vi "Kalman_Filter_Initialize.vi"(8 "error in (no error)":errorcluster, 11 "Kalman_Filter in":refnum<class "Kalman_Filter.lvclass">) -> (0 "error out":errorcluster, 3 "Kalman_Filter out":refnum<class "Kalman_Filter.lvclass">)   [LabVIEW 2021, in "Kalman_Filter.lvclass"]
uses:
  Kalman_Filter.lvclass
  Kalman_Filter.lvclass/Kalman_Filter.ctl
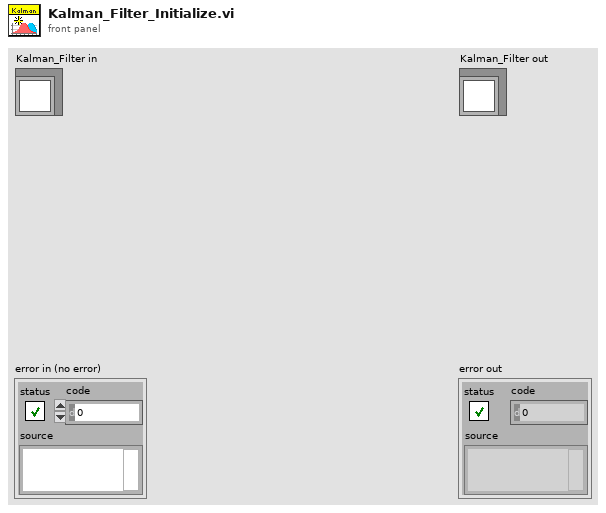
[diagram p1: front panel]
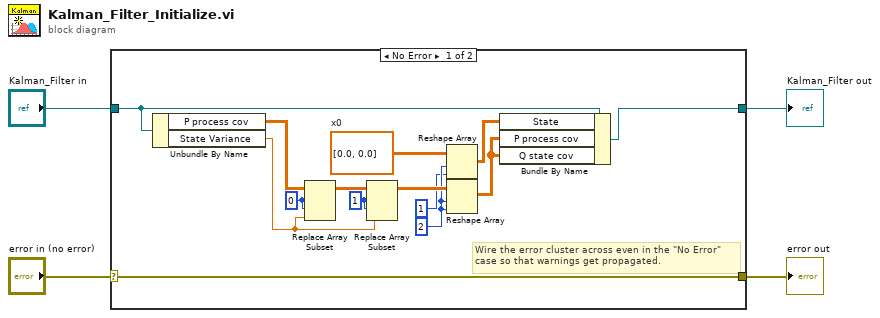
[diagram p0: block diagram]
diagram:
  n1 = case shown="No Error" "error in (no error)" {
    selector: "error in (no error)" -> [w18 w20]
    tunnel: [w18 w20] -> w3
    tunnel: [w12 w19] -> w1
    tunnel: "Kalman_Filter in" -> [w13 w19]
    frame No Error {
      w7 = 2
      w10 = 1 ("disabled index (col)")
      w8 = 0 ("index (row)")
      w17 = dbl[][] [[0.0], [0.0]]  # x0
      # "Wire the error cluster across even in the \"No Error\"\ncase so that warnings get propagated."
      n2 = Unbundle By Name(w13) -> ("P process cov"=w11:dbl[][], "State Variance"=w15:dbl)
      n3 = Replace Array Subset(array=w11, new element=w15, index (row)=w8, index (col)=w8) -> (w9:dbl[][])
      n4 = Replace Array Subset(array=w9, new element=w15, index (row)=w10, index (col)=w10) -> (w16:dbl[][])
      n5 = Reshape Array(w17, w7, 1) -> (w14:dbl[][])
      n6 = Reshape Array(w16, w7, w7) -> (w5:dbl[][])
      n7 = Bundle By Name(cluster=w13, "State"=w14, "P process cov"=w5, "Q state cov"=w5) -> (w12:refnum<class "Kalman_Filter.lvclass">)
    }
    frame Error {
    }
  }
  "error out" <- w3
  "Kalman_Filter out" <- w1
